vi "COMI PID Set Params.vi"(9 "pPidParams":T1, 10 "nNumCtrls":i32, 11 "hDevice":u32) -> (1 "pPidParams out":T1, 2 "function return":i32, 3 "hDevice out":u32)   [LabVIEW 2017, in "Comidll.lvlib"]
doc: "int (COMI_PID_SetParams) (HANDLE hDevice, int nNumCtrls, TPidParams *pPidParams);"
uses:
  <userlib>/Comidll/Comidll.lvlib
  <userlib>/Comidll/Comidll.dll
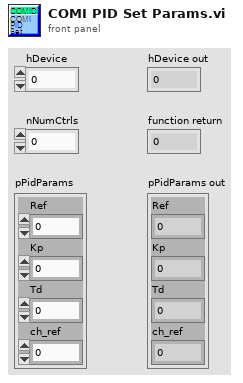
[diagram p1: front panel]
types:
  T1 = cluster{"Ref":sgl, "Kp":sgl, "Td":sgl, "ch_ref":i32}
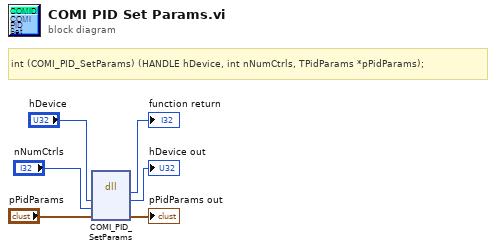
[diagram p0: block diagram]
diagram:
  # "int\t(COMI_PID_SetParams) (HANDLE hDevice, int nNumCtrls, TPidParams *pPidParams);"
  n1 = dll-call lib="C:/Program Files/National Instruments/LabVIEW 2017/user.lib/Comidll/Comidll.*" fn="COMI_PID_SetParams"("hDevice"="hDevice", "nNumCtrls"="nNumCtrls", "pPidParams"="pPidParams") -> (→"function return":i32, "hDevice"=→"hDevice out":u32, "pPidParams"=→"pPidParams out":T1)  [unwired: 4 in, 2 out]
